vi "Joystick and Camera.vi"() -> ()   [LabVIEW 2016]
uses:
  Classes/Controller/Camera/Machine Vision.ctl
  Classes/Controller/I-O/I-O.lvclass
  Classes/Controller/Motion/Motion.lvclass
  Classes/Controller/Camera/Camera.lvclass
  Classes/Controller/Controller.lvclass
panel:
  out "XYZTheta Out":dbl[](array[numeric])
  in  "Machine Vision":T1
  in  "Move 10cm Right":bool
  in  "Move 10cm Backward":bool
  in  "Move 10cm Forward":bool
  in  "Move 10cm Left":bool
  in  "Record Measurement":bool=TRUE
  in  "Dismount Silicon":bool
  in  "Dismount Silicon Tray":bool
  in  "Secure Silicon":bool
  in  "Secure Silicon Tray":bool
  in  "Z Go":bool
  in  "Position":dbl
  in  "XYZTheta":dbl[](array[numeric])
  in  "Go":bool
  in  "Joystick":bool
  out "Sum":dbl[](array[numeric])
  out "Gantry":dbl[](array[numeric])
  in  "Stop":bool
  out "Image":T2(plugin-control)
  out "Camera":dbl[](array[numeric])
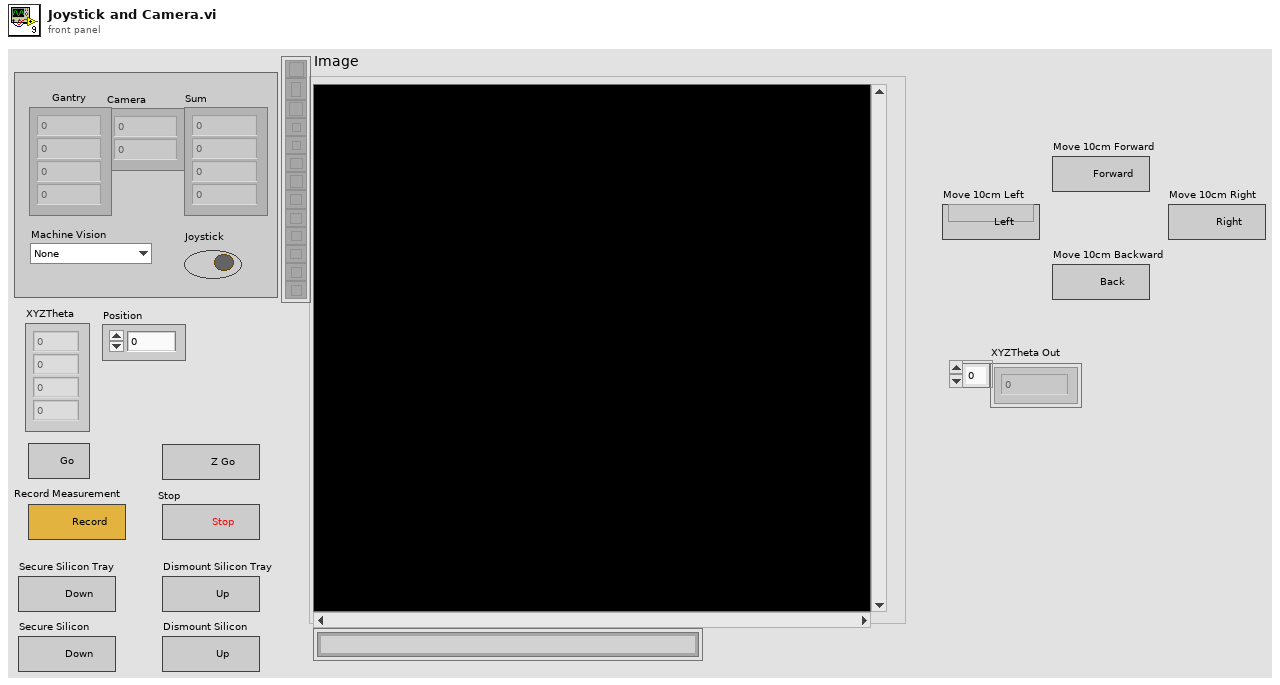
[diagram p1: front panel]
types:
  T1 = typedef "Camera.lvclass/Machine Vision.ctl" = enum16{"None", "Tray Fiducials", "HPK Silicon", "Hexaboard", "Corner (TL, BR)", "Corner (BL, TR)"}
  T2 = typedef "IMAQ Image.ctl" = refnum<image>
  T3 = typedef "Controller.lvclass/Controllers.ctl" = cluster{"I-O.lvclass":refnum<class "I-O.lvclass">, "Motion.lvclass":refnum<class "Motion.lvclass">, "Dispenser.lvclass":refnum<class "Dispenser.lvclass">}
  T4 = typedef "I-O.lvclass/Pin Map.ctl" = cluster{"Region Valves":i32[], "Extra Valves":dbl[][][], "Tool Primary Valve":i32, "Tool Secondary Valve":i32, "Region Sensors":i32[], "Extra Sensors":dbl[][][], "Tool Primary Sensor":dbl, "Tool Secondary Sensor":dbl, "Compression Sensor":dbl, "5V":i32}
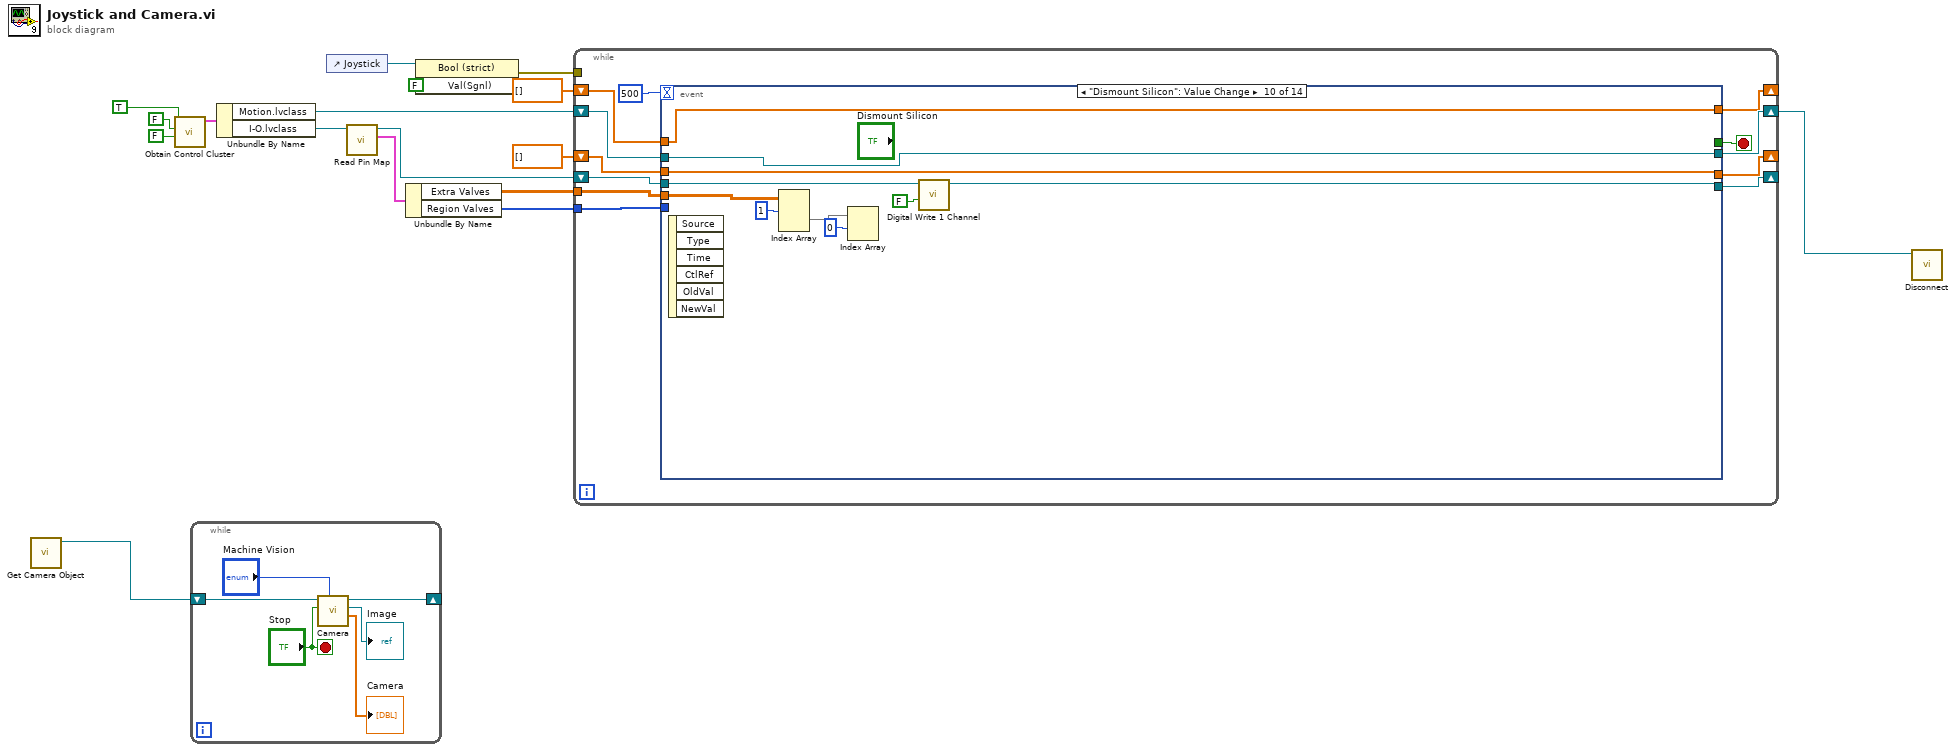
[diagram p0: block diagram]
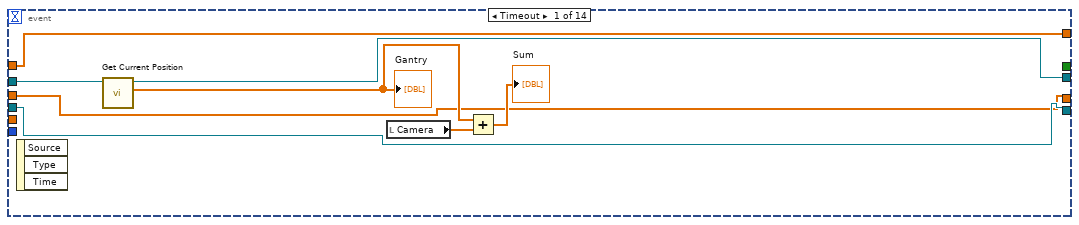
[diagram p2: hidden frame]
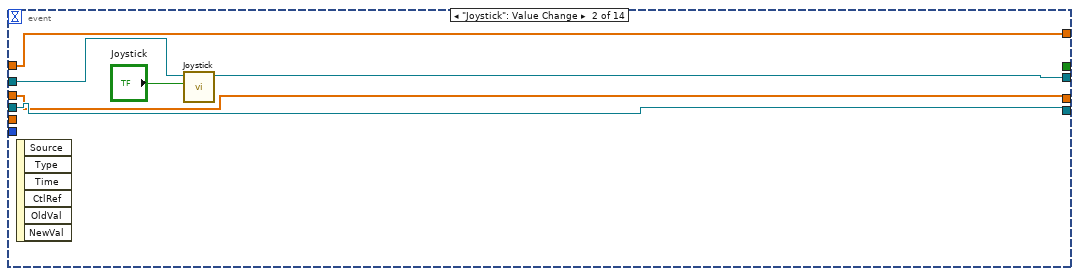
[diagram p3: hidden frame]
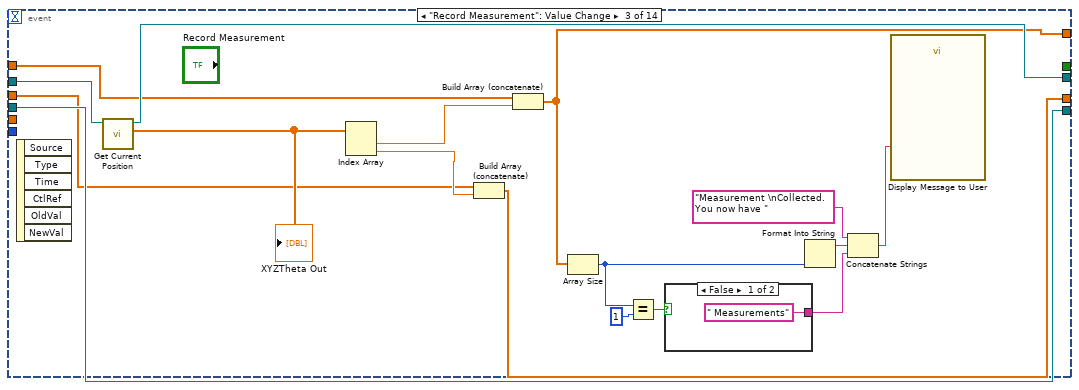
[diagram p4: hidden frame]
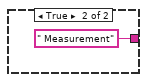
[diagram p5: hidden frame]
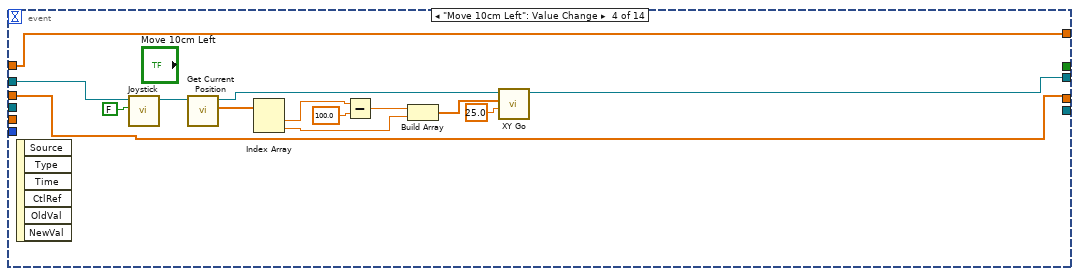
[diagram p6: hidden frame]
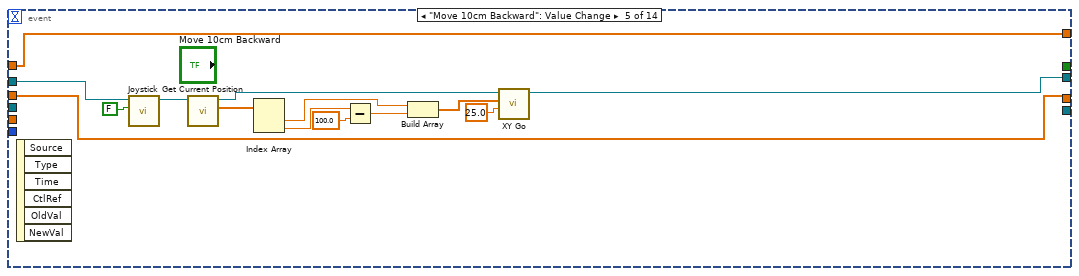
[diagram p7: hidden frame]
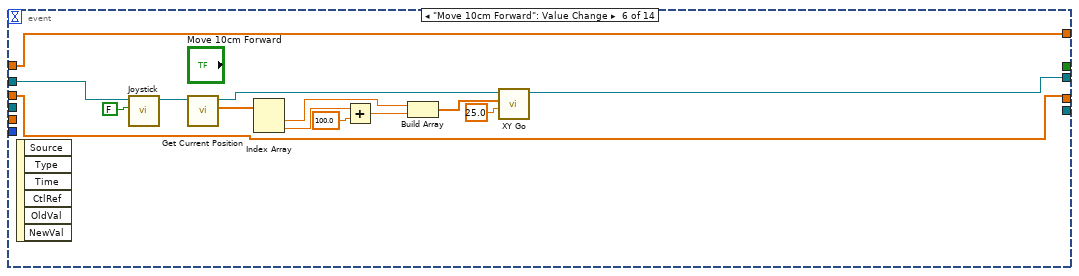
[diagram p8: hidden frame]
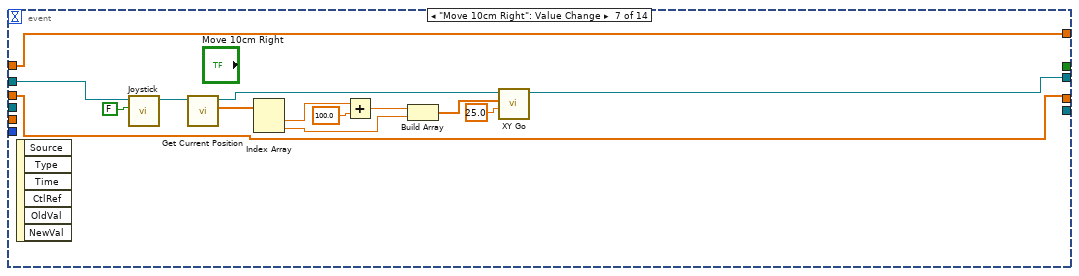
[diagram p9: hidden frame]
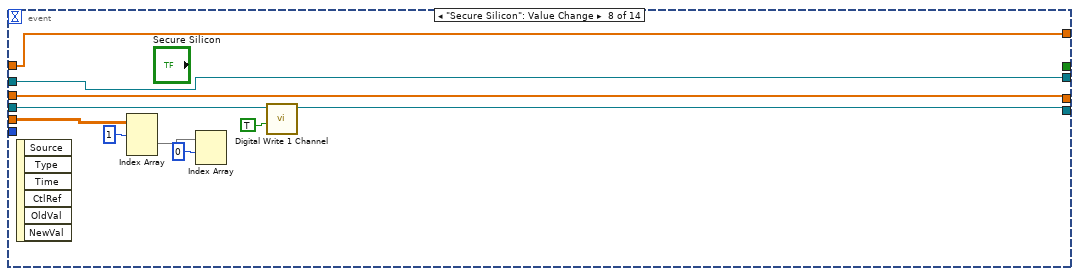
[diagram p10: hidden frame]
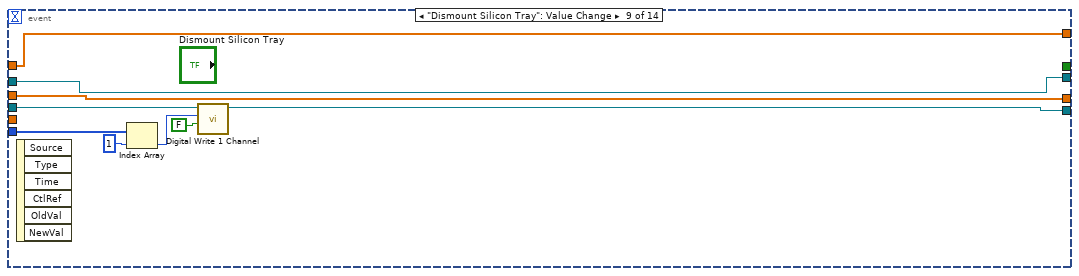
[diagram p11: hidden frame]
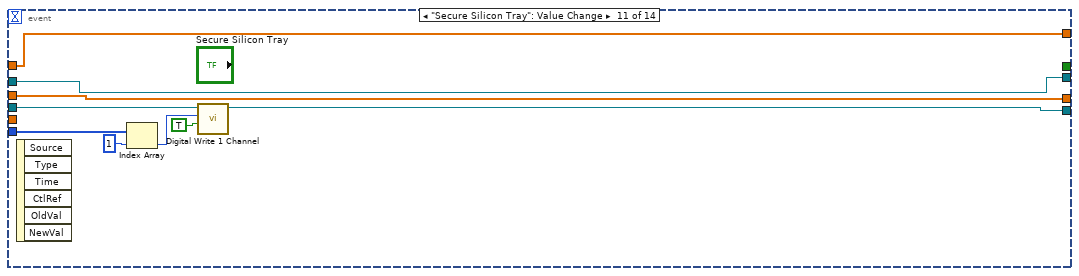
[diagram p12: hidden frame]
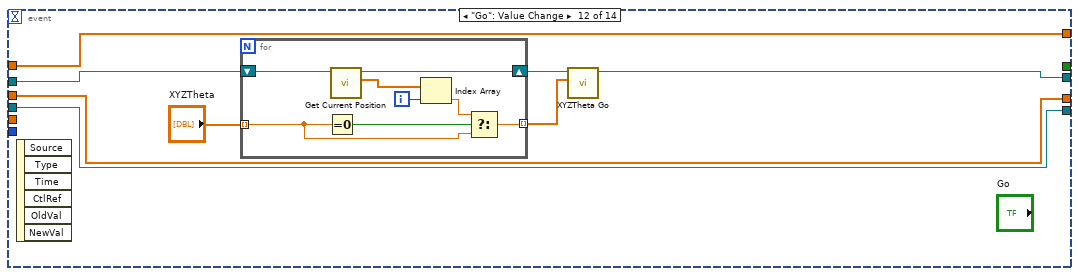
[diagram p13: hidden frame]
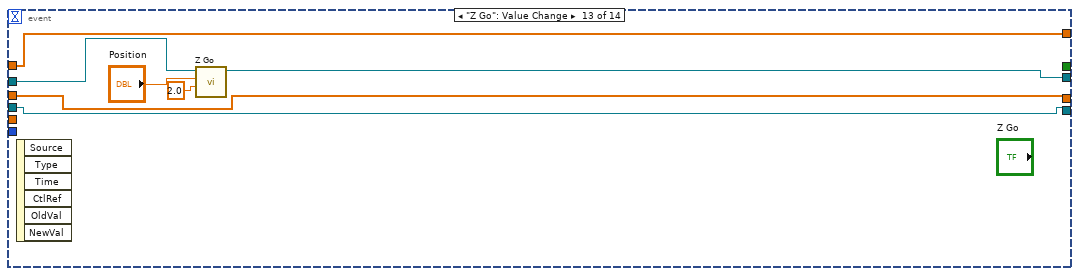
[diagram p14: hidden frame]
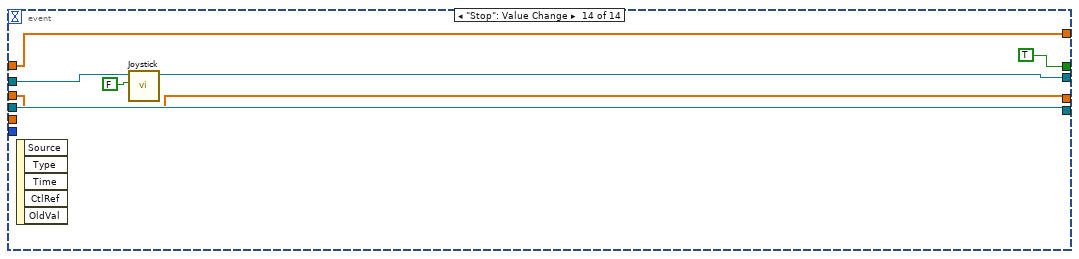
[diagram p15: hidden frame]
diagram:
  n1 = call "Get Camera Object.vi"() -> ("Camera out"=w9:refnum<class "Camera.lvclass">)  [unwired: 10 in, 1 out]
  n2 = call "Obtain Control Cluster.vi"("I/O"=FALSE, "Dispense"=FALSE, "Motion"=TRUE) -> ("Control Out"=w11:T3)  [unwired: 8 in]
  n3 = while {
    shift-right: [w22] -> _
    shift-left: w9 -> [w23]
    stop <- "Stop" stop-if-true
    n4 = call "Camera.vi"("Machine Vision"="Machine Vision", "Stop"="Stop", "Camera in"=w23) -> ("Camera"=→"Camera":dbl[], "Image"=→"Image":T2, "Camera out"=w22:refnum<class "Camera.lvclass">)  [unwired: 5 in, 1 out]
  }
  n5 = Unbundle By Name(w11) -> ("Motion.lvclass"=w10:refnum<class "Motion.lvclass">, "I-O.lvclass"=w8:refnum<class "I-O.lvclass">)
  n6 = control-ref of="Joystick"() -> (w16:refnum<vi>)
  n7 = call-dynamic "Read Pin Map.vi"("I-O in"=w8) -> ("Pin Map"=w6:T4, "I-O out"=w7:refnum<class "I-O.lvclass">)  [unwired: 8 in, 1 out]
  n8 = Unbundle By Name(w6) -> ("Extra Valves"=w4:dbl[][][], "Region Valves"=w5:i32[])
  n9 = property class="Bool (strict)"(reference=w16, "Val(Sgnl)"=FALSE ("Value (Signaling)")) -> (error out=w14:errorcluster)  [unwired: 1 in, 1 out]
  n10 = while {
    shift-right: [w32] -> w15
    shift-left: w10 -> [w33]
    tunnel: w14 -> [_]
    shift-right: [w30] -> _
    shift-left: w7 -> [w31]
    tunnel: w5 -> [w29]
    tunnel: w4 -> [w28]
    shift-right: [w25] -> _
    shift-left: dbl[] [] -> [w27]
    shift-right: [w24] -> _
    shift-left: dbl[] [] -> [w26]
    stop <- w34 stop-if-true
    n11 = event shown="[9] \"Dismount Silicon\": Value Change" {
      selector: _ -> [_ _ _ _ _ _ _ _ _ _ _ _ _ _]
      dyn-events: _ -> [_ _ _ _ _ _ _ _ _ _ _ _ _ _]
      timeout: 500 -> [_ _ _ _ _ _ _ _ _ _ _ _ _ _]
      tunnel: [_ _ _ _ _ _ _ _ _ _ _ _ _ TRUE] -> w34
      tunnel: w33 -> [w41 w49 w66 w73 w86 w100 w114 w127 w137 w146 w161 w169 w185 w191]
      tunnel: [w40 w47 w65 w74 w93 w105 w117 w127 w137 w146 w161 w166 w184 w189] -> w32
      tunnel: w31 -> [w39 w46 w64 _ _ _ _ w130 w141 w149 w162 w165 w181 w188]
      tunnel: [w39 w46 w64 _ _ _ _ w129 w138 w148 w156 w165 w181 w188] -> w30
      tunnel: w29 -> [_ _ _ _ _ _ _ _ w143 _ w160 _ _ _]
      tunnel: w28 -> [_ _ _ _ _ _ _ w134 _ w153 _ _ _ _]
      tunnel: w27 -> [w37 w45 w50 w70 w84 w98 w112 w126 w136 w145 w155 w164 w180 w187]
      tunnel: [w37 w45 w54 w70 w84 w98 w112 w126 w136 w145 w155 w164 w180 w187] -> w25
      tunnel: w26 -> [w36 w44 w51 w69 w83 w97 w111 w125 w135 w144 w154 w163 w179 w186]
      tunnel: [w36 w44 w53 w69 w83 w97 w111 w125 w135 w144 w154 w163 w179 w186] -> w24
      event Timeout {
        n12 = event-data() -> ()  [unwired: 1 in, 3 out]
        n13 = call-dynamic "Get Current Position.vi"("Motion in"=w41) -> ("XYZTheta Out"=w38:dbl[], "Motion out"=w40:refnum<class "Motion.lvclass">)  [unwired: 8 in, 1 out]
        "Gantry" <- w38
        n14 = local read "Camera"() -> (w43:dbl[])
        n15 = Add(x=w38, y=w43) -> (x+y=→"Sum":dbl[])
      }
      event "Joystick": Value Change {
        n16 = event-data() -> ()  [unwired: 1 in, 6 out]
        n17 = call-dynamic "Joystick.vi"("Joystick"="Joystick", "Motion in"=w49) -> ("Motion out"=w47:refnum<class "Motion.lvclass">)  [unwired: 8 in, 1 out]
      }
      event "Record Measurement": Value Change {
        n18 = event-data() -> ()  [unwired: 1 in, 6 out]
        n19 = call-dynamic "Get Current Position.vi"("Motion in"=w66) -> ("XYZTheta Out"=w55:dbl[], "Motion out"=w65:refnum<class "Motion.lvclass">)  [unwired: 8 in, 1 out]
        "XYZTheta Out" <- w55
        n20 = Index Array(array=w55) -> (element #1=w63:dbl, element #2=w52:dbl)  [unwired: 2 in]
        n21 = Build Array (concatenate)(w50, w52) -> (w54:dbl[])
        n22 = Build Array (concatenate) "Build Array"(w51, w63) -> (w53:dbl[])
        n23 = Array Size(array=w53) -> (size(s)=w58:i32)
        n24 = Equal?(x=w58, y=1) -> (x = y?=w57:bool)
        n25 = case shown="False" w57 {
          tunnel: [" Measurements" " Measurement"] -> w56
          frame False {
          }
          frame True {
          }
        }
        n26 = Format Into String(w58) -> (resulting string=w62:string)  [unwired: 3 in, 1 out]
        n27 = Concatenate Strings("Measurement \nCollected. You now have ", w62, w56) -> (w60:string)
        n28 = call "Display Message to User"("Message"=w60) -> ()  [unwired: 9 in, 2 out]
      }
      event "Move 10cm Left": Value Change {
        n29 = event-data() -> ()  [unwired: 1 in, 6 out]
        n30 = call-dynamic "Joystick.vi"("Joystick"=FALSE, "Motion in"=w73) -> ("Motion out"=w72:refnum<class "Motion.lvclass">)  [unwired: 8 in, 1 out]
        n31 = call-dynamic "Get Current Position.vi"("Motion in"=w72) -> ("XYZTheta Out"=w81:dbl[], "Motion out"=w82:refnum<class "Motion.lvclass">)  [unwired: 8 in, 1 out]
        n32 = Index Array(array=w81) -> (element #1=w80:dbl, element #2=w77:dbl)  [unwired: 2 in]
        n33 = Subtract(x=w80, y=100.0) -> (x-y=w78:dbl)
        n34 = Build Array(w78, w77) -> (w76:dbl[])
        n35 = call-dynamic "XY Go.vi"("Speed"=25.0, "XY"=w76, "Motion in"=w82) -> ("Motion out"=w74:refnum<class "Motion.lvclass">)  [unwired: 7 in, 1 out]
      }
      event "Move 10cm Backward": Value Change {
        n36 = event-data() -> ()  [unwired: 1 in, 6 out]
        n37 = call-dynamic "Joystick.vi"("Joystick"=FALSE, "Motion in"=w86) -> ("Motion out"=w85:refnum<class "Motion.lvclass">)  [unwired: 8 in, 1 out]
        n38 = call-dynamic "Get Current Position.vi"("Motion in"=w85) -> ("XYZTheta Out"=w95:dbl[], "Motion out"=w96:refnum<class "Motion.lvclass">)  [unwired: 8 in, 1 out]
        n39 = Index Array(array=w95) -> (element #1=w89:dbl, element #2=w92:dbl)  [unwired: 2 in]
        n40 = Subtract(x=w92, y=100.0) -> (x-y=w90:dbl)
        n41 = Build Array(w89, w90) -> (w88:dbl[])
        n42 = call-dynamic "XY Go.vi"("Speed"=25.0, "XY"=w88, "Motion in"=w96) -> ("Motion out"=w93:refnum<class "Motion.lvclass">)  [unwired: 7 in, 1 out]
      }
      event "Move 10cm Forward": Value Change {
        n43 = event-data() -> ()  [unwired: 1 in, 6 out]
        n44 = call-dynamic "Joystick.vi"("Joystick"=FALSE, "Motion in"=w100) -> ("Motion out"=w99:refnum<class "Motion.lvclass">)  [unwired: 8 in, 1 out]
        n45 = call-dynamic "Get Current Position.vi"("Motion in"=w99) -> ("XYZTheta Out"=w109:dbl[], "Motion out"=w110:refnum<class "Motion.lvclass">)  [unwired: 8 in, 1 out]
        n46 = Index Array(array=w109) -> (element #1=w103:dbl, element #2=w104:dbl)  [unwired: 2 in]
        n47 = Add(x=w104, y=100.0) -> (x+y=w102:dbl)
        n48 = Build Array(w103, w102) -> (w107:dbl[])
        n49 = call-dynamic "XY Go.vi"("Speed"=25.0, "XY"=w107, "Motion in"=w110) -> ("Motion out"=w105:refnum<class "Motion.lvclass">)  [unwired: 7 in, 1 out]
      }
      event "Move 10cm Right": Value Change {
        n50 = event-data() -> ()  [unwired: 1 in, 6 out]
        n51 = call-dynamic "Joystick.vi"("Joystick"=FALSE, "Motion in"=w114) -> ("Motion out"=w113:refnum<class "Motion.lvclass">)  [unwired: 8 in, 1 out]
        n52 = call-dynamic "Get Current Position.vi"("Motion in"=w113) -> ("XYZTheta Out"=w123:dbl[], "Motion out"=w124:refnum<class "Motion.lvclass">)  [unwired: 8 in, 1 out]
        n53 = Index Array(array=w123) -> (element #1=w116:dbl, element #2=w120:dbl)  [unwired: 2 in]
        n54 = Add(x=w116, y=100.0) -> (x+y=w121:dbl)
        n55 = Build Array(w121, w120) -> (w119:dbl[])
        n56 = call-dynamic "XY Go.vi"("Speed"=25.0, "XY"=w119, "Motion in"=w124) -> ("Motion out"=w117:refnum<class "Motion.lvclass">)  [unwired: 7 in, 1 out]
      }
      event "Secure Silicon": Value Change {
        n57 = event-data() -> ()  [unwired: 1 in, 6 out]
        n58 = Index Array(array=w134, index (dim 0)=1) -> (element=w132:dbl[][])  [unwired: 2 in]
        n59 = Index Array(array=w132, index (row)=0) -> ()  [unwired: 1 in, 1 out]
        n60 = call-dynamic "Digital Write 1 Channel.vi"("Value"=TRUE, "I-O.lvclass"=w130) -> ("I-O.lvclass 2"=w129:refnum<class "I-O.lvclass">)  [unwired: 8 in, 1 out]
      }
      event "Dismount Silicon Tray": Value Change {
        n61 = event-data() -> ()  [unwired: 1 in, 6 out]
        n62 = Index Array(array=w143, index=1) -> (element=w140:i32)
        n63 = call-dynamic "Digital Write 1 Channel.vi"("Value"=FALSE, "Channel"=w140, "I-O.lvclass"=w141) -> ("I-O.lvclass 2"=w138:refnum<class "I-O.lvclass">)  [unwired: 7 in, 1 out]
      }
      event "Dismount Silicon": Value Change {
        n64 = event-data() -> ()  [unwired: 1 in, 6 out]
        n65 = Index Array(array=w153, index (dim 0)=1) -> (element=w151:dbl[][])  [unwired: 2 in]
        n66 = Index Array(array=w151, index (row)=0) -> ()  [unwired: 1 in, 1 out]
        n67 = call-dynamic "Digital Write 1 Channel.vi"("Value"=FALSE, "I-O.lvclass"=w149) -> ("I-O.lvclass 2"=w148:refnum<class "I-O.lvclass">)  [unwired: 8 in, 1 out]
      }
      event "Secure Silicon Tray": Value Change {
        n68 = event-data() -> ()  [unwired: 1 in, 6 out]
        n69 = Index Array(array=w160, index=1) -> (element=w158:i32)
        n70 = call-dynamic "Digital Write 1 Channel.vi"("Value"=TRUE, "Channel"=w158, "I-O.lvclass"=w162) -> ("I-O.lvclass 2"=w156:refnum<class "I-O.lvclass">)  [unwired: 7 in, 1 out]
      }
      event "Go": Value Change {
        n71 = event-data() -> ()  [unwired: 1 in, 6 out]
        n72 = for {
          tunnel: "XYZTheta" -> [w176] mode=indexing
          tunnel: [w174] -> w168 mode=indexing
          shift-right: [w172] -> w167
          shift-left: w169 -> [w173]
          i -> [w178]
          n73 = Equal To 0?(x=w176) -> (x = 0?=w177:bool)
          n74 = call-dynamic "Get Current Position.vi"("Motion in"=w173) -> ("XYZTheta Out"=w171:dbl[], "Motion out"=w172:refnum<class "Motion.lvclass">)  [unwired: 8 in, 1 out]
          n75 = Index Array(array=w171, index=w178) -> (element=w175:dbl)
          n76 = Select(t=w175, s=w177, f=w176) -> (s? t:f=w174:dbl)
        }
        n77 = call "XYZTheta Go.vi"("XYZTheta In"=w168, "Motion in"=w167) -> ("Motion out"=w166:refnum<class "Motion.lvclass">)  [unwired: 7 in, 2 out]
      }
      event "Z Go": Value Change {
        n78 = event-data() -> ()  [unwired: 1 in, 6 out]
        n79 = call-dynamic "Z Go.vi"("Speed"=2.0, "Position"="Position", "Motion in"=w185) -> ("Motion out"=w184:refnum<class "Motion.lvclass">)  [unwired: 7 in, 1 out]
      }
      event "Stop": Value Change {
        n80 = event-data() -> ()  [unwired: 1 in, 5 out]
        n81 = call-dynamic "Joystick.vi"("Joystick"=FALSE, "Motion in"=w191) -> ("Motion out"=w189:refnum<class "Motion.lvclass">)  [unwired: 8 in, 1 out]
      }
    }
  }
  n82 = call-dynamic "Disconnect.vi"("Controller in"=w15) -> ()  [unwired: 9 in, 1 out]
